vi "b.vi"() -> (8 "HP34401 2":refnum<visa-resource-name>="COM1", 9 "第一路电压（V） 2":dbl=5.0, 10 "GWS 2":refnum<visa-resource-name>="COM4", 11 "第一路电流（A） 2":dbl=1.0, 12 "CONST820 2":refnum<visa-resource-name>="COM3", 13 "第二路电压（V） 2":dbl=5.0, 14 "DH1766-2 2":refnum<visa-resource-name>="COM5", 15 "第二路电流 （A） 2":dbl=1.0, 16 "恒温时间（分钟） 2":i32, 17 "温度上限（℃） 2":dbl=75.0, 18 "传感器预热时间（分钟）  2":i32, 19 "温度下限（℃）  2":dbl=-45.0, 20 "检定次数  2":i32=1, 25 "温度（℃） 2":dbl[](array[numeric]), 26 "压力设定值（KPa） 2":dbl[](array[numeric]), 27 "传感器顺序编号（从1开始） 2":dbl[](array[numeric]))   [LabVIEW 2017]
panel:
  in  "温度（℃）":dbl[](array[numeric])
  in  "传感器顺序编号（从1开始）":dbl[](array[numeric])
  in  "第二路电流 （A）":dbl=1.0
  in  "第二路电压（V）":dbl=5.0
  in  "第一路电压（V）":dbl=5.0
  in  "第一路电流（A）":dbl=1.0
  in  "检定次数":i32=1
  in  "恒温时间（分钟）":i32
  in  "传感器预热时间（分钟）":i32
  in  "温度上限（℃）":dbl=75.0
  in  "温度下限（℃）":dbl=-45.0
  in  "压力设定值（KPa）":dbl[](array[numeric])
  in  "退出":bool
  in  "保存":bool
  in  "CONST820":refnum<visa-resource-name>="COM3"
  in  "DH1766-2":refnum<visa-resource-name>="COM5"
  in  "GWS":refnum<visa-resource-name>="COM4"
  in  "HP34401":refnum<visa-resource-name>="COM1"
  # "测试设置"
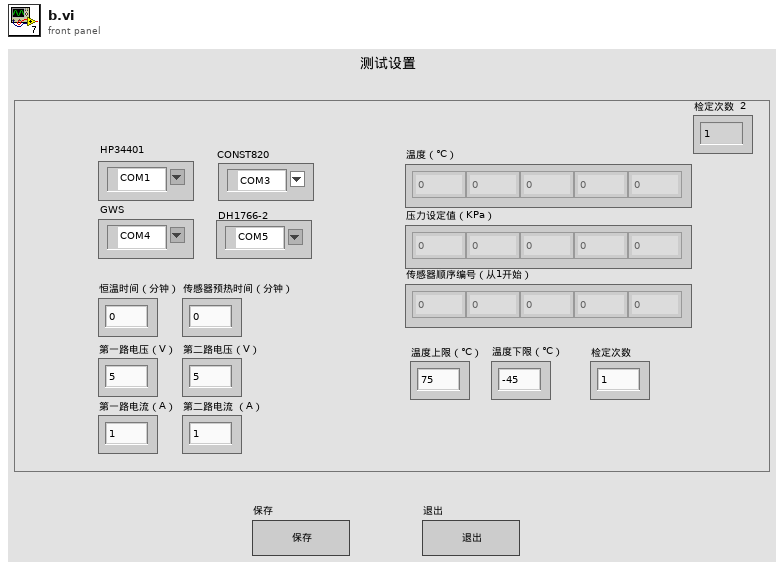
[diagram p1: front panel]
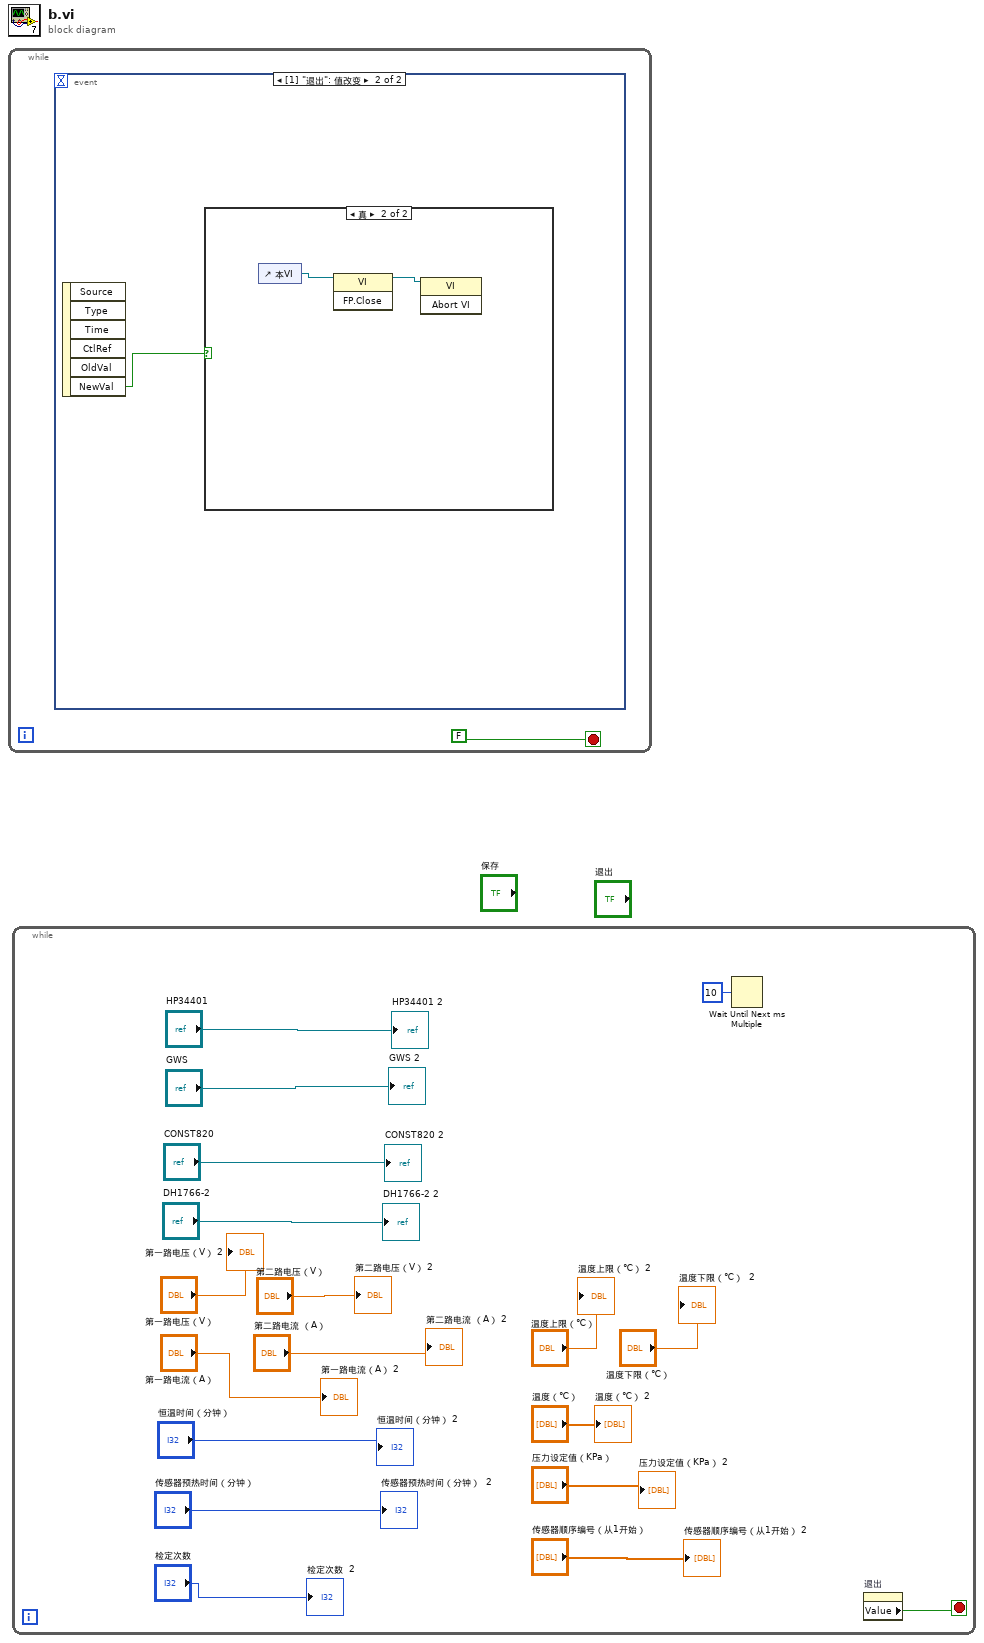
[diagram p0: block diagram]
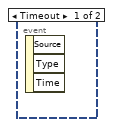
[diagram p2: hidden frame]
diagram:
  n1 = while {
    stop <- FALSE stop-if-true
    n2 = event shown="[1] \"退出\": 值改变" {
      selector: _ -> [_ _]
      dyn-events: _ -> [_ _]
      timeout: _ -> [_ _]
      event Timeout {
        n3 = event-data() -> ()  [unwired: 1 in, 3 out]
      }
      event "退出": Value Change {
        n4 = event-data() -> ("NewVal"=w2:bool)  [unwired: 1 in, 5 out]
        n5 = case shown="真" w2 {
          frame False {
          }
          frame True {
            n6 = control-ref of="本VI"() -> (w4:refnum<vi>)
            n7 = invoke class="VI" method="FP.Close"(reference=w4) -> (reference out=w3:refnum<vi>)  [unwired: 2 in, 2 out]
            n8 = invoke class="VI" method="Abort VI"(reference=w3) -> ()  [unwired: 2 in, 3 out]
          }
        }
      }
    }
  }
  n9 = while {
    stop <- w5 stop-if-true
    n10 = Wait Until Next ms Multiple(millisecond multiple=u32 10 ("毫秒倍数")) -> ()  [unwired: 1 out]
    n11 = property on="退出" class="Bool (严格)"() -> ("Value"=w5:bool)  [unwired: 2 in, 2 out]
    "HP34401 2" <- "HP34401"
    "GWS 2" <- "GWS"
    "CONST820 2" <- "CONST820"
    "DH1766-2 2" <- "DH1766-2"
    "第一路电压（V） 2" <- "第一路电压（V）"
    "第一路电流（A） 2" <- "第一路电流（A）"
    "第二路电压（V） 2" <- "第二路电压（V）"
    "第二路电流 （A） 2" <- "第二路电流 （A）"
    "恒温时间（分钟） 2" <- "恒温时间（分钟）"
    "传感器预热时间（分钟）  2" <- "传感器预热时间（分钟）"
    "温度上限（℃） 2" <- "温度上限（℃）"
    "温度下限（℃）  2" <- "温度下限（℃）"
    "温度（℃） 2" <- "温度（℃）"
    "压力设定值（KPa） 2" <- "压力设定值（KPa）"
    "传感器顺序编号（从1开始） 2" <- "传感器顺序编号（从1开始）"
    "检定次数  2" <- "检定次数"
  }
